vi "Init Device.vi"(7 "Layout Ref":refnum<vi>, 8 "error in (no error)":errorcluster, 10 "Chan# Array":i32[](array[numeric]), 11 "Aerotech_Soloist in":refnum<class "Aerotech_Soloist.lvclass">) -> (0 "error out":errorcluster, 3 "Aerotech_Soloist out":refnum<class "Aerotech_Soloist.lvclass">)   [LabVIEW 2013, in "Aerotech_Soloist.lvclass"]
doc: "Initialize the correct columns and their default appearance.\nUse the front panel to change default appearance of the device in the Add/Manage devices.\n\nOpen a specific device implementation for details."
uses:
  Aerotech_Soloist.lvclass
  TypeDefs/ColumnAppearCluster.ctl
  ColumnVIs/MenuDisableCol/MenuItemDisables.ctl
  ColumnVIs/MenuDisableCol/MenuDisableCol.lvclass
  ColumnVIs/MenuCol/MenuCol.lvclass
  ColumnVIs/Column/Column.lvclass
panel:
  in  "Name":string="AeroTech Soloist"
  in  "MenuItemDisablesList":T1[](array[typedef])=[{"MenuEntry"="IDLE", "DisableColumns"=[1, 2, 3]}, {"MenuEntry"="HOME", "DisableColumns"=[1, 2, 3]}, {"MenuEntry"="LINEAR", "DisableColumns"=[]}, {"MenuEntry"="MOVEABS", "DisableColumns"=[]}, {"MenuEntry"="MOVEINC", "DisableColumns"=[]}, {"MenuEntry"="CYCLE RESET", "DisableColumns"=[1]}]
  in  "MenuItemList":string[](array[string])=["<No Parameter Sets>"]
  in  "Device Description":string="Aerotech airstage motion controller"
  in  "Feedrate Appearance":T2={"Column Name"="Feedrate", "Width"=30, "Bkgd"=[16448250], "Text"=[0]}
  in  "Pos'n Appearance":T2={"Column Name"="Position", "Width"=30, "Bkgd"=[16448250], "Text"=[0]}
  in  "Parameters Appearance":T2={"Column Name"="Parameters", "Width"=30, "Bkgd"=[16448250], "Text"=[0]}
  in  "Command Appearance":T2={"Column Name"="Command", "Width"=30, "Bkgd"=[16448250], "Text"=[0]}
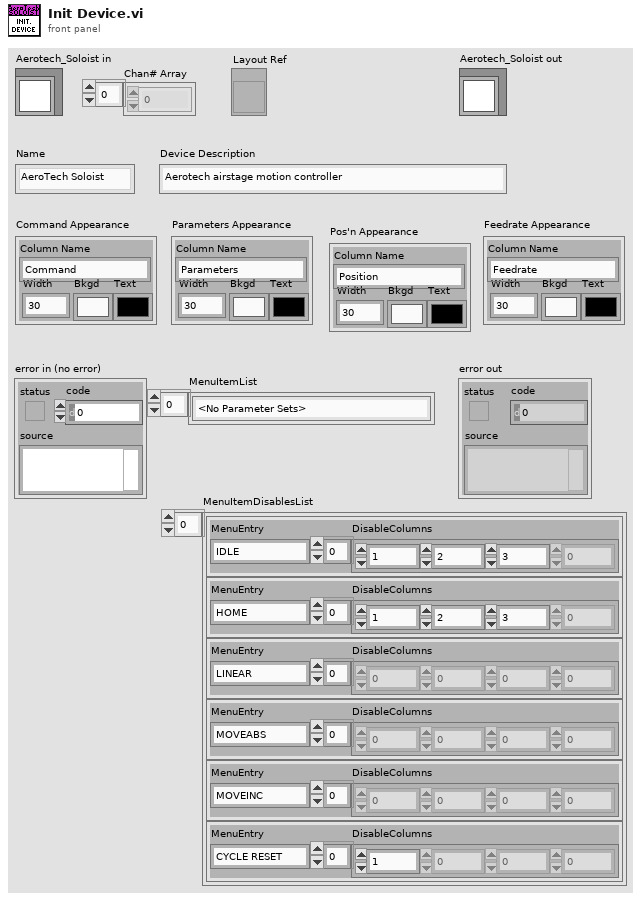
[diagram p1: front panel]
types:
  T1 = typedef "MenuItemDisables.ctl" = cluster{"MenuEntry":string, "DisableColumns":i32[]}
  T2 = typedef "ColumnAppearCluster.ctl" = cluster{"Column Name":string, "Width":u32, "Bkgd":u32[], "Text":u32[]}
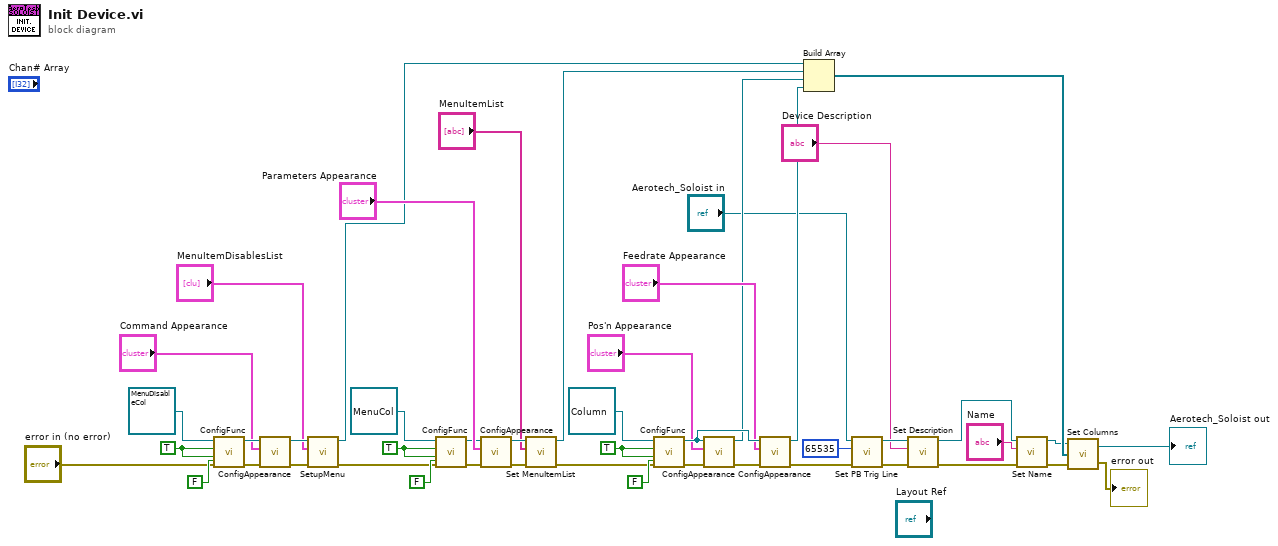
[diagram p0: block diagram]
diagram:
  w42 = TRUE ("Disableable? (True)")
  w45 = TRUE ("Disableable? (True)")
  w46 = TRUE ("Disableable? (True)")
  n1 = call "ConfigFunc.vi"("isRampable? (True"=FALSE, "error in (no error)"="error in (no error)", "isVariable? (True)"=w42, "Disableable? (True)"=w42, "Column in"=refnum<class "MenuDisableCol.lvclass"> refnum ("MenuDisableCol.lvclass")) -> ("error out"=w31:errorcluster, "Column out"=w38:refnum<class "MenuDisableCol.lvclass">)  [unwired: 5 in]
  n2 = call "ConfigAppearance.vi"("error in (no error)"=w31, "Column Appearance"="Command Appearance", "Column in"=w38) -> ("error out"=w26:errorcluster, "Column out"=w27:refnum<class "MenuDisableCol.lvclass">)  [unwired: 7 in]
  n3 = call-dynamic "SetupMenu.vi"("error in (no error)"=w26, "MenuItemDisablesList"="MenuItemDisablesList", "MenuDisableCol in"=w27) -> ("error out"=w8:errorcluster, "MenuDisableCol out"=w23:refnum<class "MenuDisableCol.lvclass">)  [unwired: 7 in]
  n4 = call "ConfigFunc.vi"("isRampable? (True"=FALSE, "error in (no error)"=w8, "isVariable? (True)"=w45, "Disableable? (True)"=w45, "Column in"=refnum<class "MenuCol.lvclass"> refnum ("MenuCol.lvclass")) -> ("error out"=w30:errorcluster, "Column out"=w35:refnum<class "MenuCol.lvclass">)  [unwired: 5 in]
  n5 = call "ConfigAppearance.vi"("error in (no error)"=w30, "Column Appearance"="Parameters Appearance", "Column in"=w35) -> ("error out"=w24:errorcluster, "Column out"=w25:refnum<class "MenuCol.lvclass">)  [unwired: 7 in]
  n6 = call-dynamic "Set MenuItemList.vi"("error in (no error)"=w24, "MenuItemList"="MenuItemList", "MenuCol in"=w25) -> ("error out"=w7:errorcluster, "MenuCol out"=w22:refnum<class "MenuCol.lvclass">)  [unwired: 7 in]
  n7 = call "ConfigFunc.vi"("isRampable? (True"=FALSE, "error in (no error)"=w7, "isVariable? (True)"=w46, "Disableable? (True)"=w46, "Column in"=refnum<class "Column.lvclass"> refnum ("Column.lvclass")) -> ("error out"=w29:errorcluster, "Column out"=w34:refnum<class "Column.lvclass">)  [unwired: 5 in]
  n8 = call "ConfigAppearance.vi"("error in (no error)"=w29, "Column Appearance"="Pos'n Appearance", "Column in"=w34) -> ("error out"=w28:errorcluster, "Column out"=w21:refnum<class "Column.lvclass">)  [unwired: 7 in]
  n9 = call "ConfigAppearance.vi"("error in (no error)"=w28, "Column Appearance"="Feedrate Appearance", "Column in"=w34) -> ("error out"=w6:errorcluster, "Column out"=w20:refnum<class "Column.lvclass">)  [unwired: 7 in]
  n10 = Build Array(w23, w22, w21, w20) -> (w19:refnum<class "Column.lvclass">[])
  n11 = call-dynamic "Set PB Trig Line.vi"("error in (no error)"=w6, "PB Trigger Line"=u16 65535, "Device in"="Aerotech_Soloist in") -> ("error out"=w14:errorcluster, "Device out"=w13:refnum<class "Aerotech_Soloist.lvclass">)  [unwired: 7 in]
  n12 = call-dynamic "Set Description.vi"("error in (no error)"=w14, "Device Description"="Device Description", "Device in"=w13) -> ("error out"=w11:errorcluster, "Device out"=w10:refnum<class "Aerotech_Soloist.lvclass">)  [unwired: 7 in]
  n13 = call-dynamic "Set Name.vi"("error in (no error)"=w11, "Name"="Name", "Device in"=w10) -> ("error out"=w15:errorcluster, "Device out"=w16:refnum<class "Aerotech_Soloist.lvclass">)  [unwired: 7 in]
  n14 = call-dynamic "Set Columns.vi"("error in (no error)"=w15, "Columns"=w19, "Device in"=w16) -> ("error out"=→"error out":errorcluster, "Device out"=→"Aerotech_Soloist out":refnum<class "Aerotech_Soloist.lvclass">)  [unwired: 1 in]
